vi "DMM Measure.vi"(8 "error in (no error)":errorcluster, 10 "SMUSequenceNumberOfSteps":i32, 11 "IVI Refnum in":refnum<k15>) -> (0 "error out":errorcluster, 1 "Numeric":dbl, 2 "Numeric 2":dbl, 3 "IVI Refnum out":refnum<k15>, 4 "Measurements":dbl[](array[numeric]))   [LabVIEW 2019]
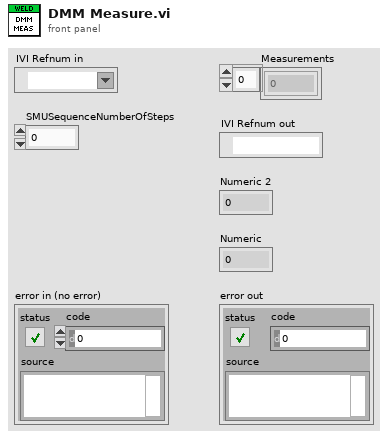
[diagram p1: front panel]
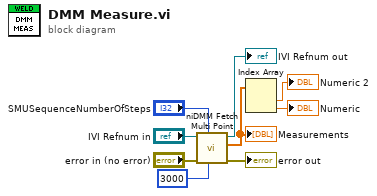
[diagram p0: block diagram]
diagram:
  n1 = call <instrlib>:"niDMM Fetch Multi Point.vi"("Maximum Time (msec)"=3000, "Number to Fetch"="SMUSequenceNumberOfSteps", "error in (no error)"="error in (no error)", "instrument handle"="IVI Refnum in") -> ("error out"=→"error out":errorcluster, "Measurements"=w6:dbl[], "instrument handle out"=→"IVI Refnum out":refnum<k15>)  [unwired: 4 in, 1 out]
  "Measurements" <- w6
  n2 = Index Array(array=w6) -> (element #1=→"Numeric 2":dbl, element #2=→"Numeric":dbl)  [unwired: 2 in]
